vi "Create plots - ring selector.vi"(6 "Relative time":bool, 7 "Data reduction":T2={"Clip time"=FALSE, "Tiime 0"=0.0, "Time 1"=0.0, "Maximum data points"=1, "Decimation method"=enum."Min-Max"}, 8 "Error In":errorcluster, 10 "File-group-channel":T1(array[cluster]), 11 "Plots  selector":cluster{"X":u16, "Y":u16}[](array[cluster]) {"Y" items=["Select channel...", "Time", "Y"]; "X" items=["Select channel...", "Time", "Y"]}) -> (0 "Error Out":errorcluster, 2 "Plots":cluster{dbl[], dbl[]}[](array[cluster]) {"?" format="%#_10g"})   [LabVIEW 2015]
uses:
  Controls/Data reduction.ctl
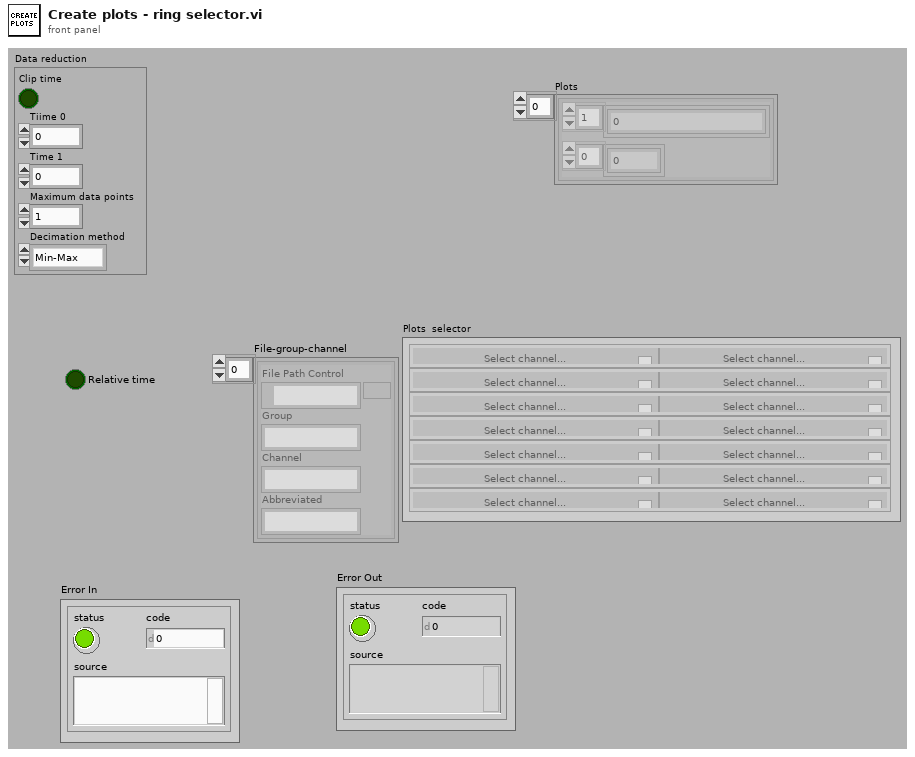
[diagram p1: front panel]
types:
  T1 = cluster{"File Path Control":path, "Group":string, "Channel":string, "Abbreviated":string}[]
  T2 = typedef "Data reduction.ctl" = cluster{"Clip time":bool, "Tiime 0":dbl, "Time 1":dbl, "Maximum data points":i32, "Decimation method":enum16{"coerce", "linear", "spline", "Min-Max", "Average"}}
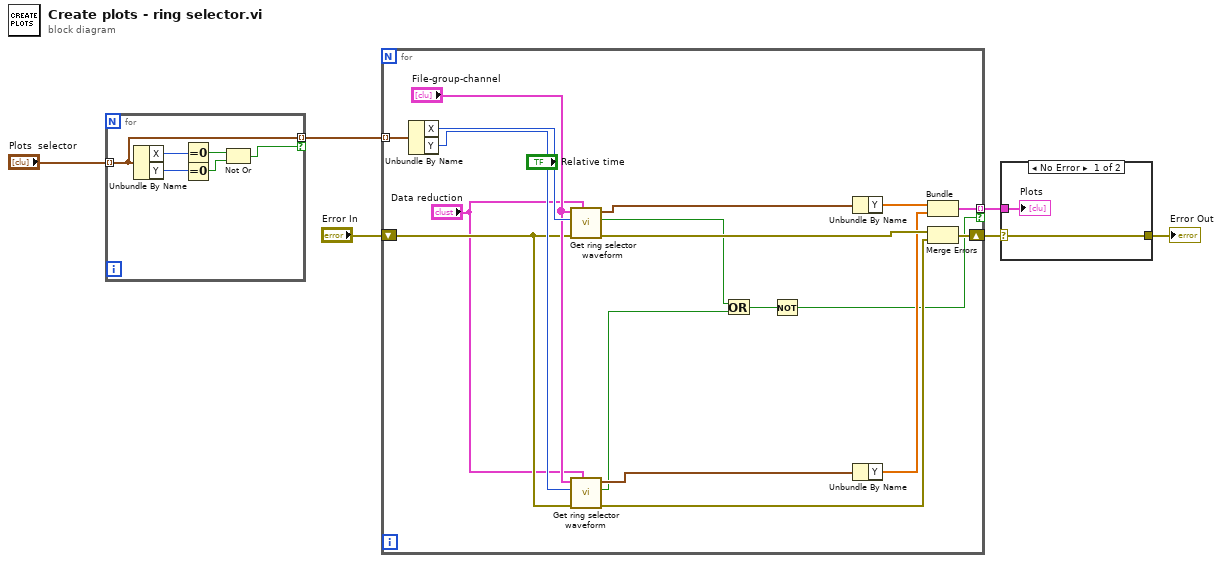
[diagram p0: block diagram]
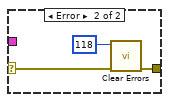
[diagram p2: hidden frame]
diagram:
  n1 = for {
    tunnel: "Plots  selector" -> [w10] mode=indexing
    tunnel: [w10] -> w5 mode=indexing if=w7
    n2 = Unbundle By Name(w10) -> ("X"=w9:u16, "Y"=w8:u16)
    n3 = Equal To 0?(x=w9) -> (x = 0?=w12:bool)
    n4 = Equal To 0?(x=w8) -> (x = 0?=w11:bool)
    n5 = Not Or(1:w11, 2:w12) -> (0:w7:bool)
  }
  n6 = for {
    tunnel: w5 -> [w30] mode=indexing
    shift-right: [w20] -> w2
    shift-left: "Error In" -> [w19]
    tunnel: [w18] -> w3 mode=indexing if=w13
    n7 = Unbundle By Name(w30) -> ("X"=w29:u16, "Y"=w28:u16)
    n8 = call "Get ring selector waveform.vi"("Clip/desimate"="Data reduction", "Error In"=w19, "Channel"=w29, "File-group-channel"="File-group-channel") -> ("Error Out"=w23:errorcluster, "Empty waveform"=w16:bool, "Waveform"=w24:waveform(sgl))  [unwired: 5 in]
    n9 = call "Get ring selector waveform.vi"("Clip/desimate"="Data reduction", "Error In"=w19, "Channel"=w28, "File-group-channel"="File-group-channel") -> ("Error Out"=w22:errorcluster, "Empty waveform"=w15:bool, "Waveform"=w25:waveform(sgl))  [unwired: 5 in]
    n10 = Or(x=w16, y=w15) -> (x .or. y?=w14:bool)
    n11 = Not(x=w14) -> (.not. x?=w13:bool)
    n12 = Unbundle By Name(w24) -> ("Y"=w26:sgl[])
    n13 = Unbundle By Name(w25) -> ("Y"=w21:sgl[])
    n14 = Bundle("Y"=w26, "Y"=w21) -> (w18:cluster{"Y":sgl[], "Y":sgl[]})  [unwired: 1 out]
    n15 = Merge Errors(w23, w22) -> (w20:errorcluster)
  }
  n16 = case shown="No Error" w2 {
    selector: w2 -> [w31 w34]
    tunnel: w3 -> [w32 _]
    tunnel: [w31 w33] -> w1
    frame No Error {
      "Plots" <- w32
    }
    frame Error {
      n17 = call <vilib>:"Clear Errors.vi"("error in (no error)"=w34, "specific error code to clear (0: all)"=118) -> ("error out"=w33:errorcluster)  [unwired: 4 in, 1 out]
    }
  }
  "Error Out" <- w1
